vi "TestExec.Config, Get Facility Info.vi"(8 "error in (no error)":errorcluster, 11 "Facility Info":path) -> (0 "error out":errorcluster, 2 "Facility Modes":path)   [LabVIEW 2018]
uses:
  <vilib>/Utility/config.llb/Read Key (String).vi
  <vilib>/Utility/config.llb/NI_LVConfig.lvlib
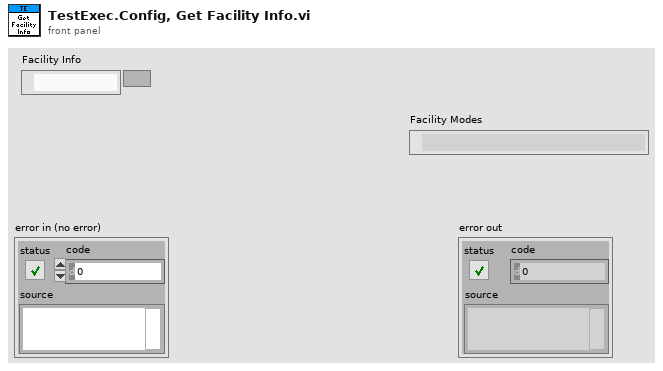
[diagram p1: front panel]
types:
  T1 = typedef "NI_LVConfig.lvlib/Config Data RefNum.ctl" = refnum<k1>
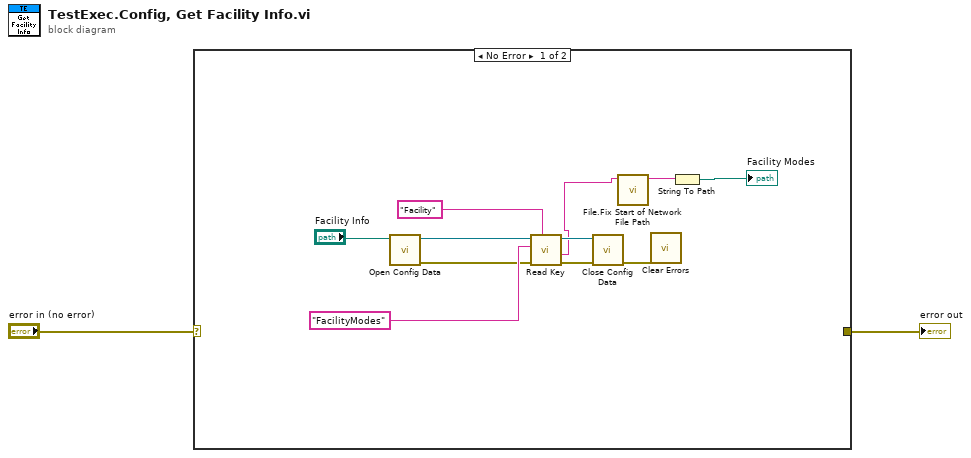
[diagram p0: block diagram]
diagram:
  n1 = case shown="No Error" "error in (no error)" {
    selector: "error in (no error)" -> [_ w14]
    tunnel: [_ w14] -> w1
    frame No Error {
      n2 = call <vilib>:"Open Config Data.vi"("configuration file path"="Facility Info") -> ("error out"=w6:errorcluster, "refnum"=w7:T1)  [unwired: 8 in, 1 out]
      n3 = call-poly <vilib>:"Read Key.vi"("section"="Facility", "error in (no error)"=w6, "key"="FacilityModes", "refnum"=w7) -> ("error out"=w11:errorcluster, "value"=w4:string, "refnum out"=w10:T1)  [unwired: 4 in, 1 out]
      n4 = call <vilib>:"Close Config Data.vi"("error in (no error)"=w11, "refnum"=w10) -> ("error out"=w12:errorcluster)  [unwired: 8 in, 1 out]
      n5 = call "File.Fix Start of Network File Path.vi"("String Path"=w4) -> ("String Path Out"=w3:string)  [unwired: 10 in]
      n6 = call <vilib>:"Clear Errors.vi"("error in (no error)"=w12) -> ()  [unwired: 5 in, 2 out]
      n7 = String To Path(string=w3) -> (path=→"Facility Modes":path)
    }
    frame Error {
    }
  }
  "error out" <- w1
